vi "CommandTranslate.vi"(0 "raw_command":u32) -> (4 "UART_Command":T1, 6 "Cmd_data":u16, 8 "UART_Ch":u8)   [LabVIEW 2015, in "UART_Firmware.lvlib"]
uses:
  UART_Firmware.lvlib
  UART_Command.ctl
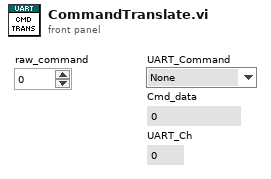
[diagram p1: front panel]
types:
  T1 = typedef "UART_Firmware.lvlib/UART_Command.ctl" = enum8{"None", "Tx", "SetBaud_High", "SetBaud_Low", "SetCharLength", "SetParity", "SetStopBits", "SetSpacing_High", "SetSpacing_Low"}
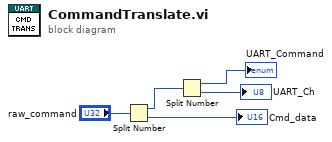
[diagram p0: block diagram]
diagram:
  n1 = Split Number(x="raw_command") -> (hi(x)=w3:u16, lo(x)=→"Cmd_data":u16)
  n2 = Split Number(x=w3) -> (hi(x)=→"UART_Command":u8, lo(x)=→"UART_Ch":u8)
